vi "Times Global.vi"() -> ()   [LabVIEW 2018]
uses:
  2019 Swerve Test Chassis/SwerveChassis2019Test 2.3/SubVis/Control 2.ctl
  2019 Swerve Test Chassis/SwerveChassis2019Test 2.3/SubVis/Control 1.ctl
  2019 Swerve Test Chassis/SwerveChassis2019Test 2.3/SubVis/Control 4.ctl
  2019 Swerve Test Chassis/SwerveChassis2019Test 2.3/SubVis/Control 3.ctl
panel:
  out "Cargo Delta Time Graph":u32(graph)
  in  "On/Off Hab Climber PT 3":bool
  in  "Hatch Panel Loop Time":T1=20.0
  in  "On/Off Hab Climber PT 2":bool
  in  "Lift Loop Time":T1=20.0
  in  "On/Off Driver Controls PT 2":bool
  in  "Manipulator Controls Loop Time":T2=20.0
  in  "On/Off Hab Climber PT":bool
  in  "On/Off Sensors PT":bool
  in  "On/Off Swerve Drive PT":bool
  in  "On/Off Driver Controls PT":bool
  in  "Hab Climber Loop Time":T1=20.0
  in  "Driver Controls Loop Time":T2=20.0
  in  "Cargo Intake Loop Time":T3=20.0
  in  "Swerve Drive Loop Time":T4=20.0
  # "Loop Times"
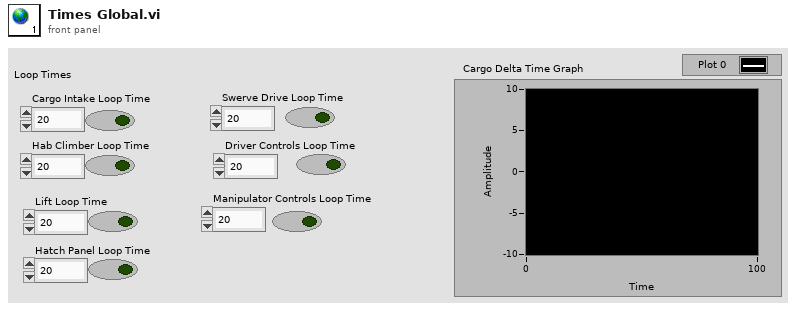
[diagram p1: front panel]
types:
  T1 = typedef "Control 3.ctl" = dbl
  T2 = typedef "Control 4.ctl" = dbl
  T3 = typedef "Control 1.ctl" = dbl
  T4 = typedef "Control 2.ctl" = dbl
diagram:
